vi "Main.vi"(10 "CaptureDetectionLoopDataIn":T1={"Period"=-1, "Reset"=TRUE, "Iteration"=0, "Capture"=path "", "Mode"={"Replay"=enum."None", "Record"=enum."None"}, "Replay Run ID"="", "Module Launched Timestamp"=timestamp(0 s since 1904-01-01), "Frame Number"=0, "Record Run ID"="", "Core Module ID"=0}, 11 "Module Admin":refnum<class "Delacor_lib_QMH_Cloneable Module Admin.lvclass">) -> ()   [LabVIEW 2026, in "UserEventRecorder.lvlib"]
doc: "This template is based off of the Queued Message Handler design pattern and the Queued Message Handler project template that ships with LabVIEW.\n\nThe main difference is that the queue is private to this module and communication between modules is performed via Broadcast and Request events.\n\nRequest events are wrapped in public API methods and are handled in the Event Handling Loop (EHL) of this VI. Any module can register for Broadcast events sent by this module. The EHL generates messages based on user interface actions.\n\nThe Message Handling Loop (MHL) processes messages generated by the EHL, or by other messages. The messages are string values, so new messages can be added easily to the Message Cases case structure in the MHL. Each message cluster can also provide an optional value for Message Data, which is a variant that can be converted to whatever message-specific data is required.\n_____\nBased on DQMH Dev Tools: Project Template 7.1.2.1547."
uses:
  UserEventRecorder.lvlib
  <vilib>/Delacor/Delacor QMH/Libraries/Cloneable Module Admin_class/Delacor_lib_QMH_Cloneable Module Admin.lvclass
  C:/Program Files/National Instruments/LabVIEW 2026/vi.lib/Delacor/Delacor QMH/Libraries/Module Admin_class/Delacor_lib_QMH_Module Admin.lvclass
  Launcher/Capture detection loop data--cluster.ctl
  Launcher/Mode.ctl
  ReplayMode.ctl
  RecordMode.ctl
  <vilib>/Wovalab/Utilities/Helper Loop Periodic Timing/Late Execution Mode--enum.ctl
  <vilib>/Wovalab/Utilities/Helper Loop Periodic Timing/Helper Loop Periodic Timing.lvclass/Helper Loop Periodic Timing.ctl
  Module Data--cluster.ctl
  <vilib>/Delacor/Delacor QMH/Libraries/Message Queue_class/Delacor_lib_QMH_Message Queue.lvclass/Delacor_lib_QMH_Message Queue.ctl
  <vilib>/Delacor/Delacor QMH/Libraries/Cloneable Module Admin_class/Delacor_lib_QMH_Cloneable Module Admin.lvclass/Delacor_lib_QMH_Cloneable Module Admin.ctl
  Stop Argument--cluster.ctl
  <vilib>/Delacor/Delacor QMH/Libraries/Module Admin_class/Delacor_lib_QMH_Module Admin.lvclass/Delacor_lib_QMH_Module Admin.ctl
  User Events Metadata.ctl
  <vilib>/Utility/miscctls.llb/LVPointTypeDef.ctl
  2c07e02c-bc34-4e84-878d-ebcb2aa1d67e.vi
  a20b1bd1-d842-476b-b4b8-d722f44d1f2b.vi
  <vilib>/Delacor/Delacor QMH/Libraries/Message Queue_class/Delacor_lib_QMH_Enqueue Message (Single).vi
  <vilib>/Delacor/Delacor QMH/Libraries/Cloneable Module Admin_class/Delacor_lib_QMH_Get Module ID.vi
  <vilib>/Delacor/Delacor QMH/Libraries/Module Admin_class/Delacor_lib_QMH_Get External Launch.vi
  <vilib>/Wovalab/Utilities/Helper Loop Periodic Timing/Stop Helper Loop Internal.vi
  <vilib>/Wovalab/Utilities/Helper Loop Periodic Timing/U32 Max Value--constant.vi
  <vilib>/Wovalab/Utilities/Helper Loop Periodic Timing/Update Last Execution Time.vi
  <vilib>/Wovalab/Utilities/Helper Loop Periodic Timing/Loops Events AE.vi
  <vilib>/Wovalab/Utilities/Helper Loop Periodic Timing/Notify Monitoring Window.vi
  <vilib>/Wovalab/Utilities/Helper Loop Periodic Timing/Monitoring--global.vi
  <userlib>/_OpenG.lib/comparison/comparison.llb/U32 Changed__ogtk.vi
  <vilib>/JDP Science/JSONtext/Variant to JSON Text.vi
  <vilib>/Wovalab/Utilities/Helper Loop Periodic Timing/Helper Loop Periodic Timing.lvclass
  <vilib>/JDP Science/JSONtext/LVClass Serializer/JSONtext LVClass Serializer.lvclass
  <vilib>/Delacor/Delacor QMH/Libraries/Message Queue_class/Delacor_lib_QMH_Message Queue.lvclass
  Launcher/Launcher.lvlib
  User32.dll
  <userlib>/_OpenG.lib/comparison/comparison.llb/openg_comparison__ogtk.lvlib
panel:
  out "Deficit":u32
  out "Frame Number":u32
  out "element 2":i32
  out "element":i32
  out "x != 0? 2":bool
  out "x != 0?":bool
  out "error out":errorcluster
  out "Status":string
  in  "Simulate EHL Error":bool
  in  "Simulate MHL Error":bool
  # "Other processes communicate with this Module via its Public API (wrappers for its Request Events).\n\nThis Module communicates with other processes via its Broadcast Events.\nAny process that wants to receive these messages can register for this module's Broadcast events."
  # "This template is for the DQMH framework. See the block diagram for more information on how to use this template."
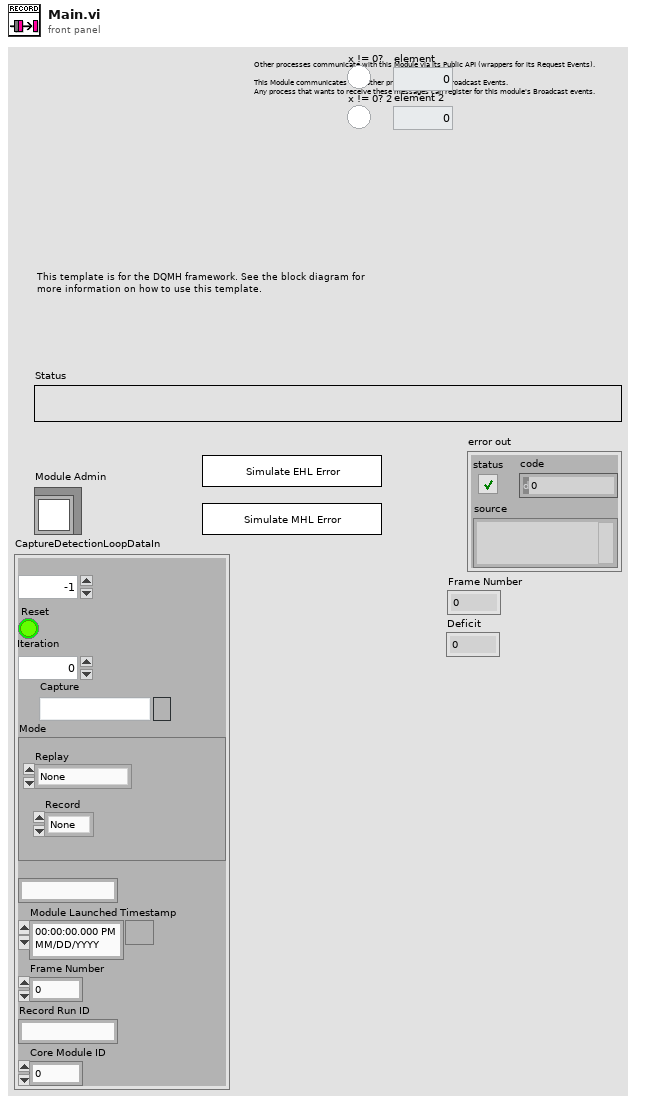
[diagram p1: front panel]
types:
  T1 = typedef "Capture detection loop data--cluster.ctl" = cluster{"Period":i32, "Reset":bool, "Iteration":i32, "Capture":path, "Mode":T2, "Replay Run ID":string, "Module Launched Timestamp":timestamp, "Frame Number":u32, "Record Run ID":string, "Core Module ID":i32}
  T2 = typedef "Mode.ctl" = cluster{"Replay":T3, "Record":T4}
  T3 = typedef "ReplayMode.ctl" = enum16{"None", "User Events"}
  T4 = typedef "RecordMode.ctl" = enum16{"None", "User Events", "Benchmarks", "User Events and Benchmarks"}
  T5 = typedef "Wovalab_lib_Utilities.lvlib/Helper Loop Periodic Timing.lvclass/Late Execution Mode--enum.ctl" = enum16{"No change", "Process missed periods ignoring original phase", "Process missed periods maintaining original phase"}
  T6 = typedef "UserEventRecorder.lvlib/Request Events--cluster.ctl" = cluster{"Stop Module":refnum<user-event>, "Show Panel":refnum<user-event>, "Hide Panel":refnum<user-event>, "Show Diagram":refnum<user-event>, "Get Module Execution Status":refnum<user-event>, "Record Frame Mouse Metadata":refnum<user-event>}
  T7 = typedef "Launcher.lvlib/Broadcast Events--cluster.ctl" = cluster{"Module Did Init":refnum<user-event>, "Status Updated":refnum<user-event>, "Error Reported":refnum<user-event>, "Module Did Stop":refnum<user-event>, "Update Module Execution Status":refnum<user-event>, "Start Capture Detection Loop":refnum<user-event>, "Benchmark Started":refnum<user-event>, "Broadcast number of frames and run ID":refnum<user-event>}
  T8 = typedef "UserEventRecorder.lvlib/Module Data--cluster.ctl" = cluster{"Status":string}
  T9 = typedef "User Events Metadata.ctl" = cluster{"Cursor Position X":i32, "Cursor Position Y":i32, "Left Button Click":bool, "Right Button Click":bool, "Frame Number":u32}
  T10 = enum16{"open", "replace", "create", "open or create", "replace or create", "replace or create with confirmation"}
  T11 = enum32{"invalid lock state", "Not Locked", "Locked (No Password)", "Password-protected"}
  T12 = typedef "UserEventRecorder.lvlib/Stop Argument--cluster.ctl" = cluster{"Module ID":i32, "Origin":string, "Exit via Stop Module Req?":bool, "Wait for Module to stop?":bool}
  T13 = typedef "LVPointTypeDef.ctl" = cluster{"Horizontal":i16, "Vertical":i16}
  T14 = enum32{"Invalid", "Standard", "Closed", "Hidden", "Minimized", "Maximized"}
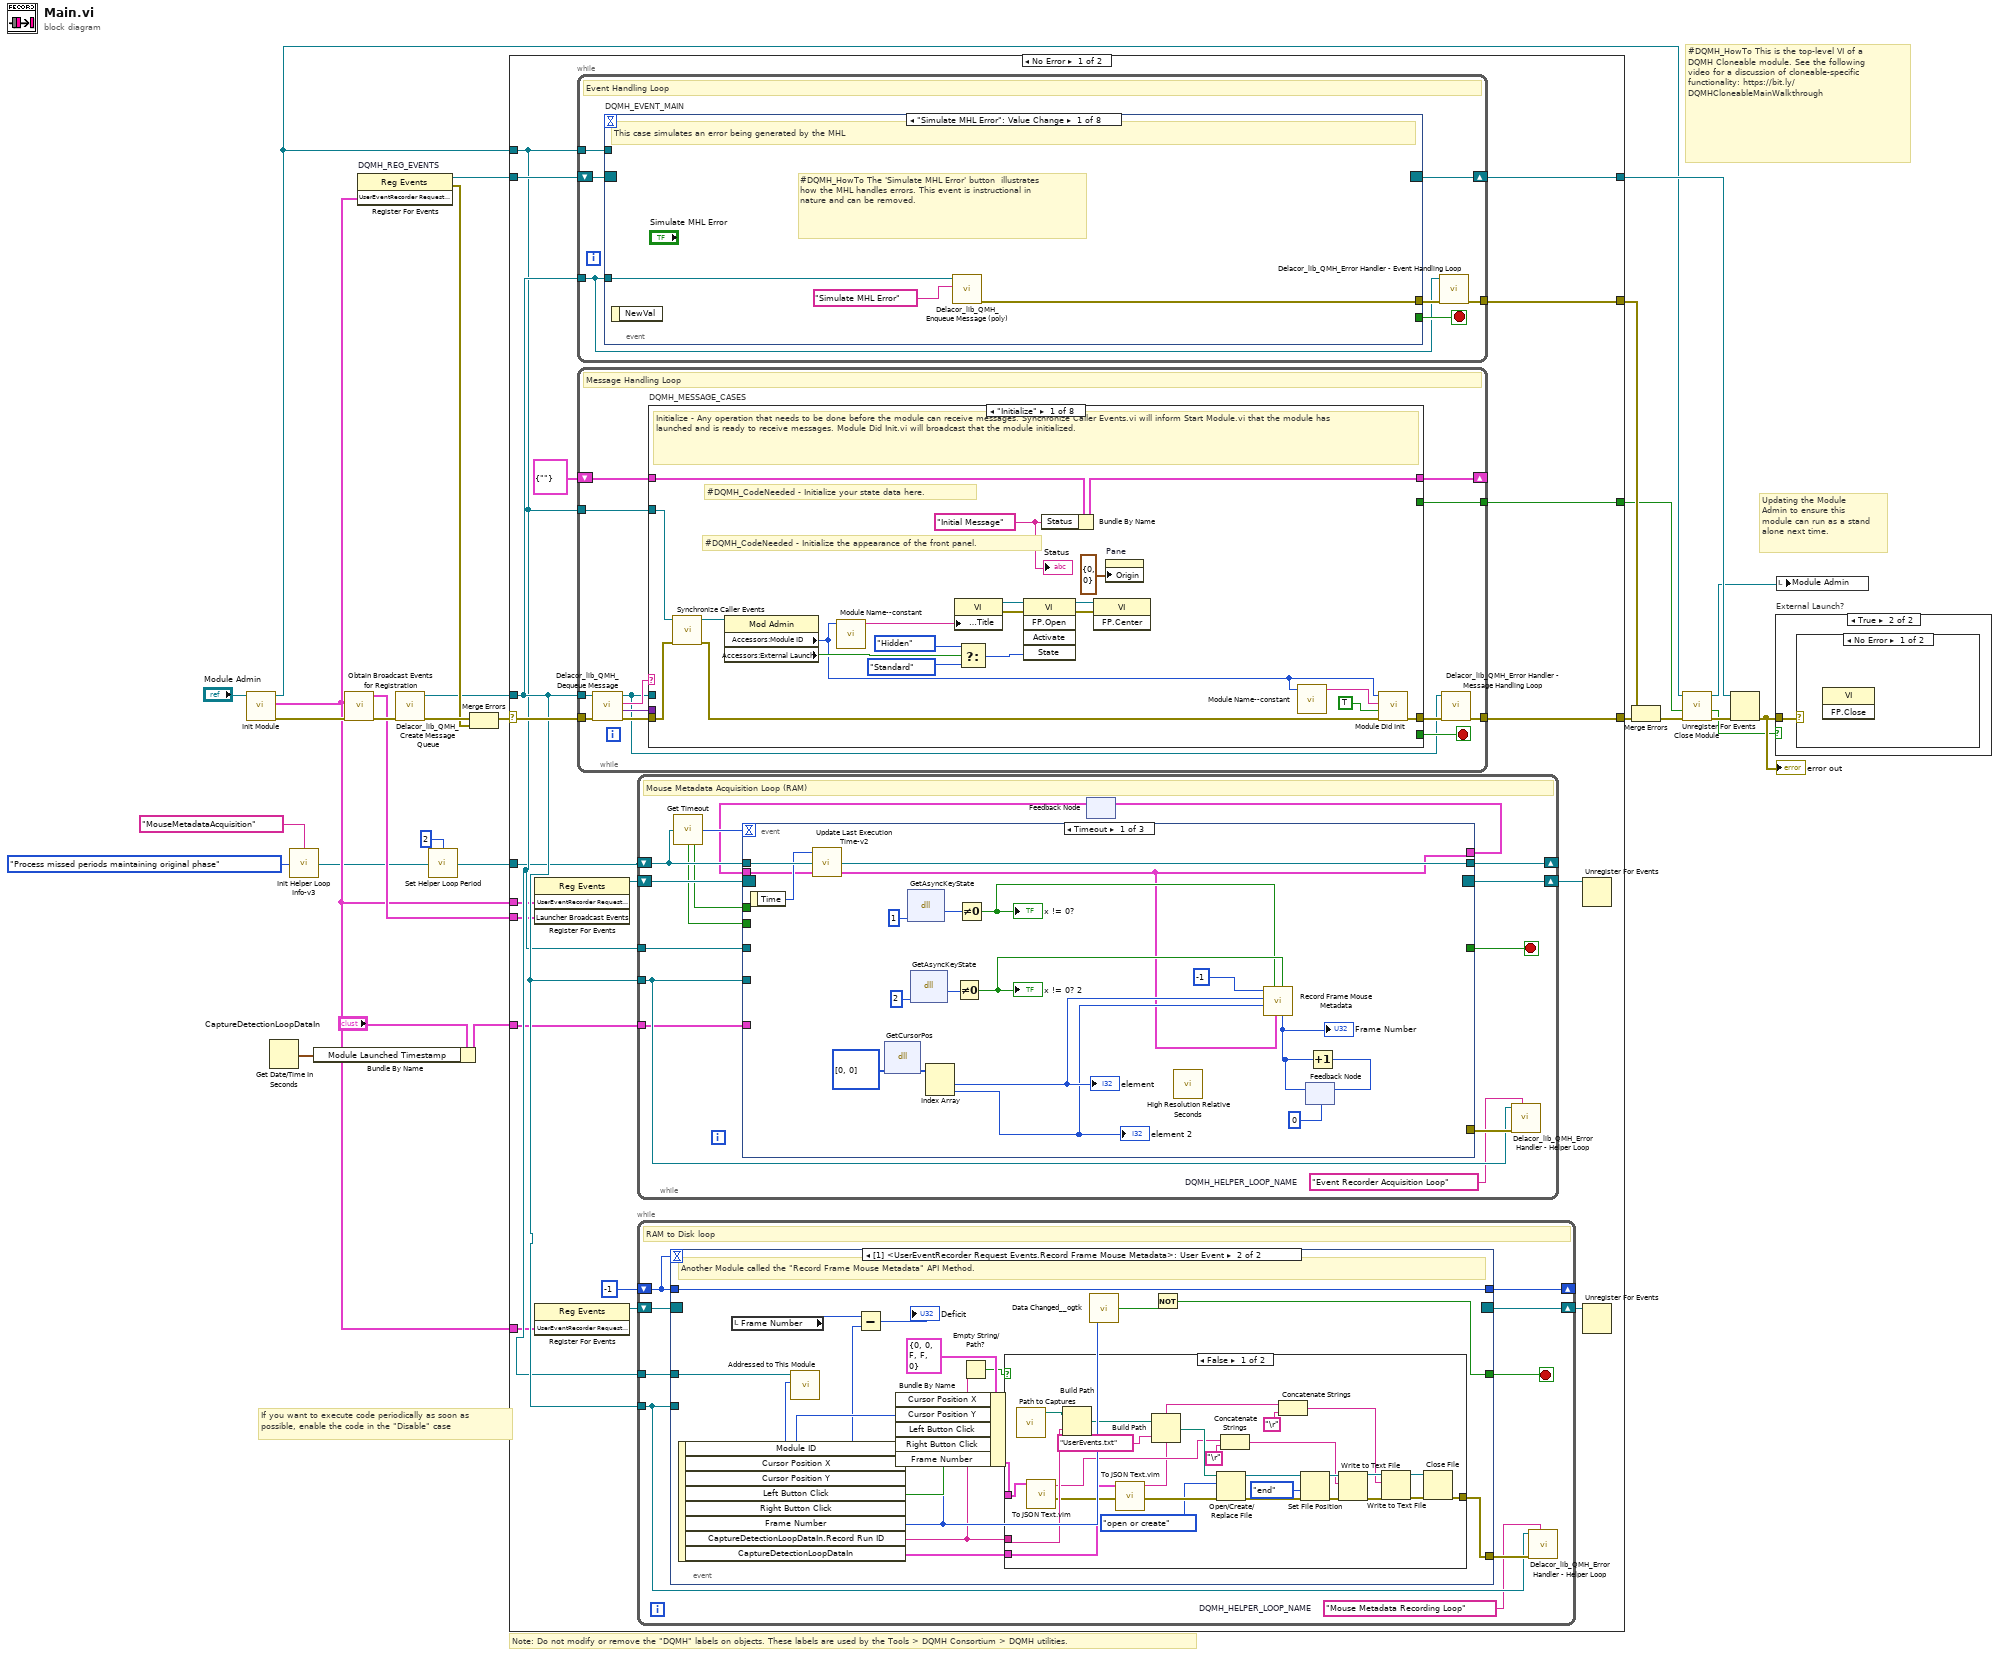
[diagram p0: block diagram]
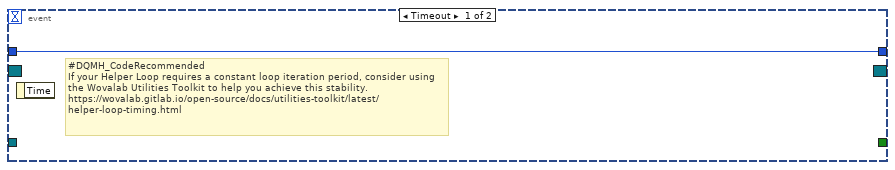
[diagram p2: hidden frame]
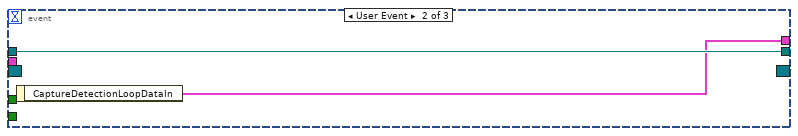
[diagram p4: hidden frame]
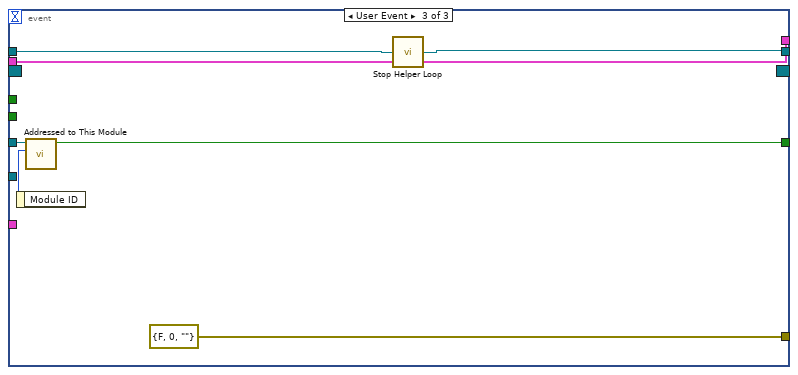
[diagram p5: hidden frame]
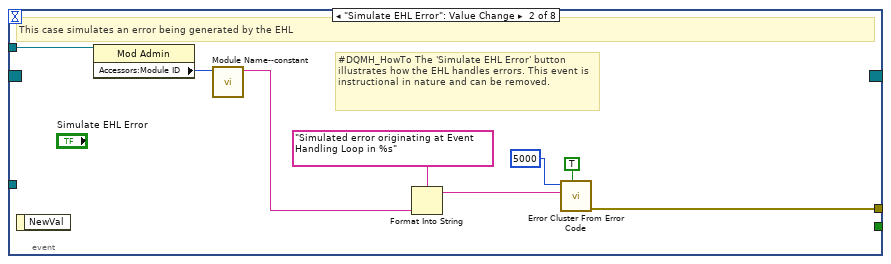
[diagram p6: hidden frame]
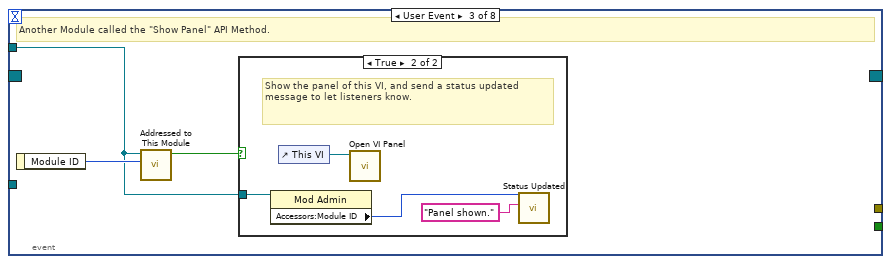
[diagram p7: hidden frame]
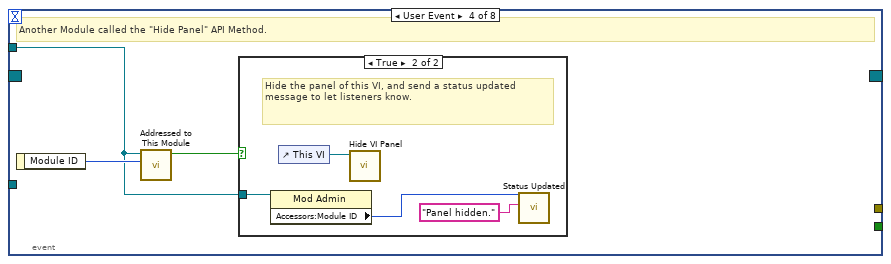
[diagram p9: hidden frame]
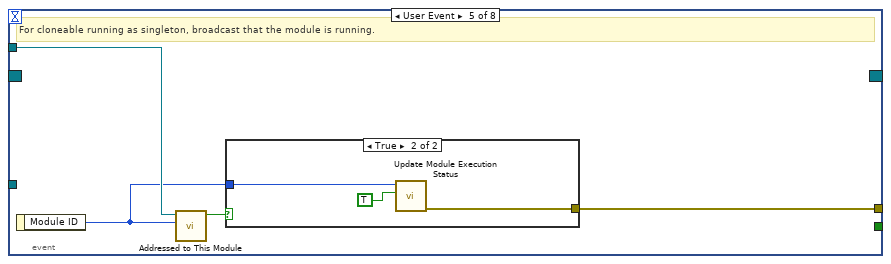
[diagram p11: hidden frame]
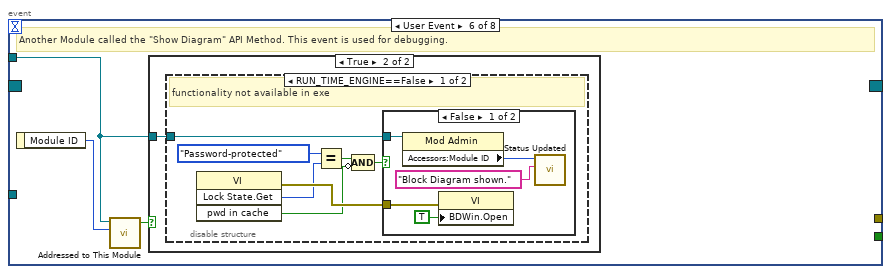
[diagram p13: hidden frame]
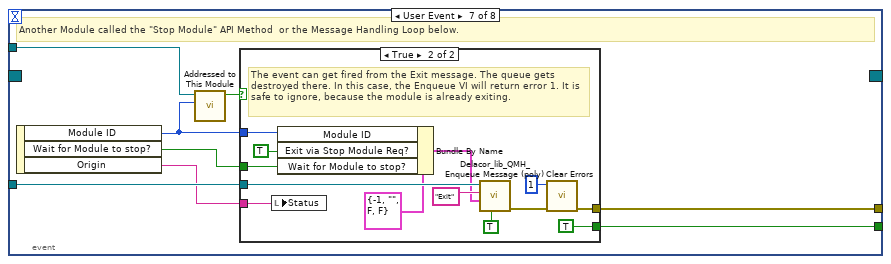
[diagram p17: hidden frame]
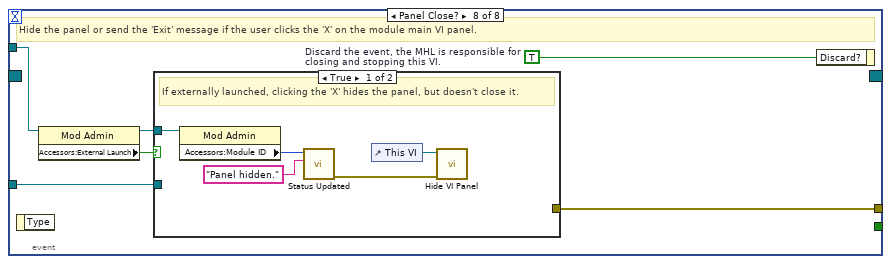
[diagram p19: hidden frame]
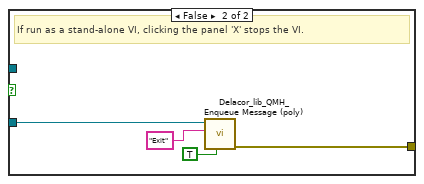
[diagram p20: hidden frame]
diagram:
  # "If you want to execute code periodically as soon as possible, enable the code in the \"Disable\" case"
  # "#DQMH_HowTo This is the top-level VI of a DQMH Cloneable module. See the following video for a discussion of cloneable-specific functionality: https://bit.ly/DQMHCloneableMainWalkthrough"
  # "Note: Do not modify or remove the \"DQMH\" labels on objects. These labels are used by the Tools > DQMH Consortium > DQMH utilities."
  # "Updating the Module Admin to ensure this module can run as a stand alone next time."
  n1 = call "Init Module.vi"("Cloneable Module Admin in"="Module Admin") -> ("error out"=w12:errorcluster, "UserEventRecorder Request Events"=w9:T6, "Cloneable Module Admin out"=w16:refnum<class "Delacor_lib_QMH_Cloneable Module Admin.lvclass">)  [unwired: 8 in]
  n2 = Get Date/Time In Seconds() -> (seconds since 1Jan1904=w1:timestamp)
  n3 = call <vilib>:"Init Helper Loop Info-v3.vi"("Late Execution Mode (Process missed periods ignoring original phase)"=Late_Execution_Mode--enum."Process missed periods maintaining original phase", "Loop Name (\"\": Caller VI)"="MouseMetadataAcquisition" ("Loop Name (\"\": Caller VI)")) -> ("Helper Loop Periodic Timing"=w5:refnum<class "Helper Loop Periodic Timing.lvclass">)
  n4 = Bundle By Name(cluster="CaptureDetectionLoopDataIn", "Module Launched Timestamp"=w1) -> (w2:T1)
  n5 = call "Obtain Broadcast Events for Registration.vi"("error in"=w12) -> ("error out"=w11:errorcluster, "Launcher Broadcast Events"=w10:T7)  [unwired: 8 in, 1 out]
  n6 = register-events "DQMH_REG_EVENTS"(w9) -> (reference out=w19:refnum<event-registration>, error out=w21:errorcluster)  [unwired: 2 in]
  n7 = call <vilib>:"Delacor_lib_QMH_Create Message Queue.vi"("error in"=w11) -> ("error out"=w23:errorcluster, "Message Queue"=w18:refnum<class "Delacor_lib_QMH_Message Queue.lvclass">)  [unwired: 9 in]
  n8 = call <vilib>:"Set Helper Loop Period.vi"("Period (ms)"=2, "Helper Loop Periodic Timing in"=w5) -> ("Helper Loop Periodic Timing out"=w4:refnum<class "Helper Loop Periodic Timing.lvclass">)  [unwired: 13 in]
  n9 = Merge Errors(w23, w21) -> (w22:errorcluster)
  n10 = case shown="No Error" w22 {
    selector: w22 -> [w45 w342]
    tunnel: [w47 w341] -> w26
    tunnel: [w44 w340] -> w20
    tunnel: w19 -> [w42 w340]
    tunnel: w18 -> [w41 w333]
    tunnel: [w46 _] -> w27
    tunnel: w16 -> [w40 w336]
    tunnel: [w39 _] -> w14
    tunnel: w9 -> [w38 _]
    tunnel: w10 -> [w35 _]
    tunnel: w9 -> [w34 _]
    tunnel: w4 -> [w30 _]
    tunnel: w2 -> [w29 _]
    frame No Error {
      n11 = register-events ("DQMH_HELPER_REGFOREVENTS")(w38, w35) -> (reference out=w36:refnum<event-registration>)  [unwired: 2 in, 1 out]
      n12 = register-events ("DQMH_HELPER_REGFOREVENTS")(w34) -> (reference out=w32:refnum<event-registration>)  [unwired: 2 in, 1 out]
      n13 = while {
        tunnel: w41 -> [w143]
        shift-right: [w146] -> w44
        shift-left: w42 -> [w147]
        tunnel: [w148] -> w46
        tunnel: w40 -> [w144]
        stop <- w145 stop-if-true
        # "Event Handling Loop"
        n14 = event "DQMH_EVENT_MAIN" shown="[0] \"Simulate MHL Error\": Value Change" {
          selector: w147 -> [_ _ _ _ _ _ _ _]
          dyn-events: [_ _ _ _ _ _ _ _] -> w146
          timeout: _ -> [_ _ _ _ _ _ _ _]
          tunnel: [_ _ _ _ _ _ w201 _] -> w145
          tunnel: w143 -> [w151 _ _ _ _ _ w204 w221]
          tunnel: [w152 w160 _ _ w178 _ w205 w224] -> w149
          tunnel: w144 -> [_ w159 w161 w168 w176 w182 w203 w222]
          event "Simulate MHL Error": Value Change {
            # "#DQMH_HowTo The 'Simulate MHL Error' button  illustrates how the MHL handles errors. This event is instructional in nature and can be removed."
            # "This case simulates an error being generated by the MHL"
            n15 = event-data() -> ()  [unwired: 1 in, 1 out]
            n16 = call-poly <vilib>:"Delacor_lib_QMH_Enqueue Message (poly).vi"("Message"="Simulate MHL Error", "Message Queue in"=w151) -> ("error out"=w152:errorcluster)  [unwired: 8 in, 1 out]
          }
          event "Simulate EHL Error": Value Change {
            # "#DQMH_HowTo The 'Simulate EHL Error' button  illustrates how the EHL handles errors. This event is instructional in nature and can be removed."
            # "This case simulates an error being generated by the EHL"
            n17 = event-data() -> ()  [unwired: 1 in, 1 out]
            n18 = property on="Property Node" class="Mod Admin"(reference=w159) -> ("Accessors:Module ID"=w158:i32)  [unwired: 1 in, 2 out]
            n19 = call "Module Name--constant.vi"("Module ID"=w158) -> ("Module Name"=w153:string)  [unwired: 10 in]
            n20 = Format Into String(format string="Simulated error originating at Event Handling Loop in %s", w153) -> (resulting string=w156:string)  [unwired: 2 in, 1 out]
            n21 = call <vilib>:"Error Cluster From Error Code.vi"("show call chain? (False)"=TRUE, "error message (\"\")"=w156, "error code (0)"=5000) -> ("error out"=w160:errorcluster)  [unwired: 6 in]
          }
          event User Event {
            # "Another Module called the \"Show Panel\" API Method."
            n22 = event-data() -> ("Module ID"=w162:i32)  [unwired: 1 in]
            n23 = call "Addressed to This Module.vi"("Module ID from Argument"=w162, "Module Admin"=w161) -> ("Addressed to this instance?"=w163:bool)  [unwired: 8 in, 1 out]
            n24 = case shown="True" w163 {
              tunnel: w161 -> [_ w165]
              frame False {
              }
              frame True {
                # "Show the panel of this VI, and send a status updated message to let listeners know."
                n25 = property on="Property Node" class="Mod Admin"(reference=w165) -> ("Accessors:Module ID"=w164:i32)  [unwired: 1 in, 2 out]
                n26 = control-ref of="This VI"() -> (w167:refnum<vi>)
                n27 = call "Open VI Panel.vi"("VI"=w167) -> ()  [unwired: 10 in, 1 out]
                n28 = call "Status Updated.vi"("Status"="Panel shown." ("format string"), "Module ID"=w164) -> ()  [unwired: 9 in, 1 out]
              }
            }
          }
          event User Event {
            # "Another Module called the \"Hide Panel\" API Method."
            n29 = event-data() -> ("Module ID"=w169:i32)  [unwired: 1 in]
            n30 = call "Addressed to This Module.vi"("Module ID from Argument"=w169, "Module Admin"=w168) -> ("Addressed to this instance?"=w170:bool)  [unwired: 8 in, 1 out]
            n31 = case shown="True" w170 {
              tunnel: w168 -> [_ w172]
              frame False {
              }
              frame True {
                # "Hide the panel of this VI, and send a status updated message to let listeners know."
                n32 = property on="Property Node" class="Mod Admin"(reference=w172) -> ("Accessors:Module ID"=w171:i32)  [unwired: 1 in, 2 out]
                n33 = control-ref of="This VI"() -> (w174:refnum<vi>)
                n34 = call "Hide VI Panel.vi"("VI"=w174) -> ()  [unwired: 10 in, 1 out]
                n35 = call "Status Updated.vi"("Status"="Panel hidden." ("format string"), "Module ID"=w171) -> ()  [unwired: 9 in, 1 out]
              }
            }
          }
          event User Event {
            # "For cloneable running as singleton, broadcast that the module is running."
            n36 = event-data() -> ("Module ID"=w175:i32)  [unwired: 1 in]
            n37 = call "Addressed to This Module.vi"("Module ID from Argument"=w175, "Module Admin"=w176) -> ("Addressed to this instance?"=w177:bool)  [unwired: 8 in, 1 out]
            n38 = case shown="True" w177 {
              tunnel: [_ w181] -> w178
              tunnel: w175 -> [_ w180]
              frame False {
              }
              frame True {
                n39 = call "Update Module Execution Status.vi"("Running?"=TRUE, "Module ID"=w180) -> ("error out"=w181:errorcluster)  [unwired: 9 in]
              }
            }
          }
          event User Event {
            # "Another Module called the \"Show Diagram\" API Method. This event is used for debugging."
            n40 = event-data() -> ("Module ID"=w183:i32)  [unwired: 1 in]
            n41 = call "Addressed to This Module.vi"("Module ID from Argument"=w183, "Module Admin"=w182) -> ("Addressed to this instance?"=w184:bool)  [unwired: 8 in, 1 out]
            n42 = case shown="True" w184 {
              tunnel: w182 -> [_ w185]
              frame False {
              }
              frame True {
                n43 = disable-structure shown="RUN_TIME_ENGINE==False" {
                  disable-tunnel: w185 -> [w186 _]
                  frame condition #0 (active) {
                    # "functionality not available in exe"
                    n44 = invoke on="Invoke Node" class="VI" method="Lock State.Get"() -> (error out=w192:errorcluster, "Get Lock State"=w191:T11, "pwd in cache"=w188:bool)  [unwired: 4 in, 1 out]
                    n45 = Equal?(x=T11."Password-protected", y=w191) -> (x = y?=w189:bool)
                    n46 = Compound Arithmetic op=AND(w189, invert w188) -> (w187:bool)
                    n47 = case shown="False" w187 {
                      tunnel: w192 -> [w197 _]
                      tunnel: w186 -> [w194 _]
                      frame False {
                        n48 = property on="Property Node" class="Mod Admin"(reference=w194) -> ("Accessors:Module ID"=w193:i32)  [unwired: 1 in, 2 out]
                        n49 = property on="Property Node" class="VI"(error in=w197, "BDWin.Open"=TRUE ("Block Diagram Window:Open")) -> ()  [unwired: 1 in, 2 out]
                        n50 = call "Status Updated.vi"("Status"="Block Diagram shown." ("format string"), "Module ID"=w193) -> ()  [unwired: 9 in, 1 out]
                      }
                      frame True {
                        # "Password-protected VI, and the password is not in the cache. Do not show the diagram."
                      }
                    }
                  }
                  frame condition #1 {
                  }
                }
              }
            }
          }
          event User Event {
            # "Another Module called the \"Stop Module\" API Method  or the Message Handling Loop below."
            n51 = event-data() -> ("Module ID"=w199:i32, "Wait for Module to stop?"=w200:bool, "Origin"=w198:string)  [unwired: 1 in]
            n52 = call "Addressed to This Module.vi"("Module ID from Argument"=w199, "Module Admin"=w203) -> ("Addressed to this instance?"=w202:bool)  [unwired: 8 in, 1 out]
            n53 = case shown="True" w202 {
              tunnel: [_ w217] -> w205
              tunnel: w204 -> [_ w213]
              tunnel: [_ TRUE] -> w201
              tunnel: w200 -> [_ w208]
              tunnel: w199 -> [_ w210]
              tunnel: w198 -> [_ w206]
              frame False {
              }
              frame True {
                # "The event can get fired from the Exit message. The queue gets destroyed there. In this case, the Enqueue VI will return error 1. It is safe to ignore, because the module is already exiting."
                n54 = local write "Status"(w206) -> ()
                n55 = Bundle By Name(cluster=T12 {"Module ID"=-1, "Origin"="", "Exit via Stop Module Req?"=FALSE, "Wait for Module to stop?"=FALSE} ("Stop Argument"), "Module ID"=w210, "Exit via Stop Module Req?"=TRUE, "Wait for Module to stop?"=w208) -> (w207:T12)
                n56 = call-poly <vilib>:"Delacor_lib_QMH_Enqueue Message (poly).vi"("Priority Message? (F)"=TRUE, "Message Data"=w207, "Message"="Exit", "Message Queue in"=w213) -> ("error out"=w218:errorcluster)  [unwired: 6 in, 1 out]
                n57 = call <vilib>:"Clear Errors.vi"("error in (no error)"=w218, "specific error code to clear (0: all)"=1) -> ("error out"=w217:errorcluster)  [unwired: 4 in, 1 out]
              }
            }
          }
          event Panel Close? {
            w223 = TRUE  # Discard the event, the MHL is responsible for closing and stopping this VI.
            # "Hide the panel or send the 'Exit' message if the user clicks the 'X' on the module main VI panel."
            n58 = event-data() -> ()  [unwired: 1 in, 1 out]
            n59 = property on="Property Node" class="Mod Admin"(reference=w222) -> (reference out=w219:refnum<class "Delacor_lib_QMH_Cloneable Module Admin.lvclass">, "Accessors:External Launch"=w220:bool)  [unwired: 1 in, 1 out]
            n60 = case shown="True" w220 {
              tunnel: w221 -> [_ w232]
              tunnel: [_ w233] -> w224
              tunnel: w219 -> [w227 _]
              frame True {
                # "If externally launched, clicking the 'X' hides the panel, but doesn't close it."
                n61 = property on="Property Node" class="Mod Admin"(reference=w227) -> ("Accessors:Module ID"=w226:i32)  [unwired: 1 in, 2 out]
                n62 = call "Status Updated.vi"("Status"="Panel hidden." ("format string"), "Module ID"=w226) -> ("error out"=w225:errorcluster)  [unwired: 9 in]
                n63 = control-ref of="This VI"() -> (w229:refnum<vi>)
                n64 = call "Hide VI Panel.vi"("error in"=w225, "VI"=w229) -> ()  [unwired: 9 in, 1 out]
              }
              frame False {
                # "If run as a stand-alone VI, clicking the panel 'X' stops the VI."
                n65 = call-poly <vilib>:"Delacor_lib_QMH_Enqueue Message (poly).vi"("Priority Message? (F)"=TRUE, "Message"="Exit", "Message Queue in"=w232) -> ("error out"=w233:errorcluster)  [unwired: 7 in, 1 out]
              }
            }
            n66 = event-data ("Event Filter Node")("Discard?"=w223) -> ()  [unwired: 1 in, 1 out]
          }
        }
        n67 = call-dynamic "Delacor_lib_QMH_Error Handler - Event Handling Loop.vi"("error in"=w149, "Message Queue in"=w143) -> ("dup error in"=w148:errorcluster)  [unwired: 8 in, 1 out]
      }
      n68 = while {
        tunnel: w41 -> [w234]
        shift-right: [w241] -> _
        shift-left: T8 {"Status"=""} ("Data Cluster") -> [w242]
        tunnel: w45 -> [w245]
        tunnel: [w243] -> w47
        tunnel: w40 -> [w236]
        tunnel: [w235] -> w39
        stop <- w240 stop-if-true
        # "Message Handling Loop"
        n69 = call-dynamic "Delacor_lib_QMH_Dequeue Message.vi"("error in"=w245, "Message Queue in"=w234) -> ("error out"=w244:errorcluster, "Message Data"=w238:variant, "Message"=w239:string, "Message Queue out"=w237:refnum<class "Delacor_lib_QMH_Message Queue.lvclass">)  [unwired: 6 in]
        n70 = case "DQMH_MESSAGE_CASES" shown="\"Initialize\"" w239 {
          selector: w239 -> [_ _ _ _ _ _ _ w322]
          tunnel: w237 -> [_ _ _ _ w277 _ w314 _]
          tunnel: w244 -> [w265 w269 w272 w274 w286 w303 w320 w331]
          tunnel: [w263 w269 w271 w274 w282 w302 w315 w332] -> w246
          tunnel: w242 -> [w256 w268 w270 w273 w281 w300 w313 w329]
          tunnel: [w255 w268 w270 w273 w281 w300 w313 w329] -> w241
          tunnel: [_ _ _ _ _ _ w312 _] -> w240
          tunnel: w238 -> [_ _ _ _ w280 _ w310 _]
          tunnel: w236 -> [w251 _ _ _ w279 w298 w305 w328]
          tunnel: [_ _ _ _ _ _ w308 _] -> w235
          frame "Initialize" {
            w248 = "Initial Message" ("Initial Message")
            # "#DQMH_CodeNeeded - Initialize the appearance of the front panel."
            # "#DQMH_CodeNeeded - Initialize your state data here."
            # "Initialize - Any operation that needs to be done before the module can receive messages. Synchronize Caller Events.vi will inform Start Module.vi that the module has launched and is ready to receive messages. Module Did Init.vi will broadcast that the module initialized."
            n71 = call "Synchronize Caller Events.vi"("error in"=w265, "Module Admin"=w251) -> ("error out"=w264:errorcluster, "Module Admin out"=w250:refnum<class "Delacor_lib_QMH_Cloneable Module Admin.lvclass">)  [unwired: 8 in]
            n72 = property on="Property Node" class="Mod Admin"(reference=w250) -> ("Accessors:Module ID"=w247:i32, "Accessors:External Launch"=w252:bool)  [unwired: 1 in, 2 out]
            n73 = call "Module Name--constant.vi"("Module ID"=w247) -> ("Module Name"=w260:string)  [unwired: 10 in]
            n74 = property on="Property Node" class="VI"("Front Panel.Title"=w260) -> (reference out=w262:refnum<vi>, error out=w267:errorcluster)  [unwired: 2 in]
            n75 = Select(t=T14."Hidden" ("State"), s=w252, f=T14."Standard" ("State")) -> (s? t:f=w257:T14)
            n76 = invoke on="Invoke Node" class="VI" method="FP.Open"(reference=w262, error in=w267, "State"=w257) -> (reference out=w261:refnum<vi>, error out=w266:errorcluster)  [unwired: 2 in, 3 out]
            n77 = Bundle By Name(cluster=w256, "Status"=w248) -> (w255:T8)
            n78 = invoke on="Invoke Node" class="VI" method="FP.Center"(reference=w261, error in=w266) -> ()  [unwired: 1 in, 3 out]
            n79 = property on="Pane" class="Pane"("Origin"=T13 {"Horizontal"=0, "Vertical"=0}) -> ()  [unwired: 2 in, 2 out]
            n80 = call "Module Name--constant.vi"("Module ID"=w247) -> ("Module Name"=w253:string)  [unwired: 10 in]
            n81 = call "Module Did Init.vi"("error in"=w264, "Initialized?"=TRUE, "Origin"=w253, "Module ID"=w247) -> ("error out"=w263:errorcluster)  [unwired: 7 in]
            "Status" <- w248
          }
          frame "---Module Specific---" {
            # "Separator -- The following cases handle messages specific to this Module."
          }
          frame "---Copy This Frame---" {
            # "Duplicate this frame when creating new messages.  Change this comment in the duplicated frame to describe this message."
            n82 = Merge Errors(w272) -> (w271:errorcluster)
          }
          frame "---Exit and Error Handling---" {
            # "Separator - the following cases handle errors and exit messages."
          }
          frame "Error" {
            # "#DQMH_CodeRecommended - If the module is running in standalone mode (External Launch = FALSE), this code will pop up an error dialog and call the 'Exit' message if an error occurs. Add more fine-grained error management here."
            # "Error - Check the error message data and respond accordingly. This message is sent by the \"Error Handler\" VIs at the end of each loop in this application."
            n83 = property on="Property Node" class="Mod Admin"(reference=w279) -> ("Accessors:External Launch"=w278:bool, "Accessors:Module ID"=w276:i32)  [unwired: 1 in, 2 out]
            n84 = Variant To Data(error in=w286, type=errorcluster {"status"=FALSE, "code"=0, "source"=""} ("error constant"), Variant=w280) -> (data=w275:errorcluster, error out=w284:errorcluster)
            n85 = local write "error out"(w275) -> ()
            n86 = call "Error Reported.vi"("Error"=w275, "Module ID"=w276) -> ()  [unwired: 9 in, 1 out]
            n87 = case shown="False" w278 {
              tunnel: [w291 _] -> w283
              tunnel: w277 -> [w289 _]
              tunnel: w275 -> [w290 _]
              frame False {
                n88 = disable-structure shown="Default" {
                  disable-tunnel: w290 -> [w292 _]
                  frame condition #0 (active) {
                    # "If the module is running standalone, then pop up an error dialog and call the \"Exit\" message."
                    n89 = call <vilib>:"Simple Error Handler.vi"("error in (no error)"=w292) -> ()  [unwired: 4 in, 5 out]
                  }
                  frame condition #1 {
                    # "To prevent the Simple Error Handler VI from being loaded (e.g. when deploying to a Real-Time target), add the Conditional Disable Symbol \"DQMH_Disable_SEH\" to your project and set it to TRUE."
                  }
                }
                n90 = call-poly <vilib>:"Delacor_lib_QMH_Enqueue Message (poly).vi"("Priority Message? (F)"=TRUE, "Message"="Exit", "Message Queue in"=w289) -> ("error out"=w291:errorcluster)  [unwired: 7 in, 1 out]
              }
              frame True {
                # "If the module was launched externally, calling the Error Reported broadcast VI is the only action performed by the \"Error\" message. The module's caller can then process the error appropriately."
              }
            }
            n91 = Merge Errors(w284, w283) -> (w282:errorcluster)
          }
          frame "Simulate MHL Error" {
            # "#DQMH_HowTo The 'Simulate MHL Error' button  illustrates how the MHL handles errors. This event is instructional in nature and can be removed."
            # "Simulate an error occurring at the MHL"
            n92 = property on="Property Node" class="Mod Admin"(reference=w298) -> ("Accessors:Module ID"=w299:i32)  [unwired: 1 in, 2 out]
            n93 = call "Module Name--constant.vi"("Module ID"=w299) -> ("Module Name"=w294:string)  [unwired: 10 in]
            n94 = Format Into String(format string="Simulated error originating at Message Handling Loop in %s", w294) -> (resulting string=w295:string)  [unwired: 2 in, 1 out]
            n95 = call <vilib>:"Error Cluster From Error Code.vi"("show call chain? (False)"=TRUE, "error message (\"\")"=w295, "error code (0)"=5001) -> ("error out"=w301:errorcluster)  [unwired: 6 in]
            n96 = Merge Errors(w303, w301) -> (w302:errorcluster)
          }
          frame "Exit" {
            w311 = 91  # 91: not all Exit messages will have an argument
            w312 = TRUE  # Stop the VI
            # "Release the message queue reference"
            # "#DQMH_CodeNeeded - Add any required cleanup code here."
            # "Exit - Exit the application."
            n97 = Variant To Data(error in=w320, type=T12 {"Module ID"=-1, "Origin"="", "Exit via Stop Module Req?"=FALSE, "Wait for Module to stop?"=FALSE} ("Stop Argument"), Variant=w310) -> (data=w307:T12, error out=w316:errorcluster)
            n98 = call <vilib>:"Clear Errors.vi"("error in (no error)"=w316, "specific error code to clear (0: all)"=w311) -> ("error out"=w319:errorcluster)  [unwired: 4 in, 1 out]
            n99 = property on="Property Node" class="Mod Admin"(reference=w305) -> ("Accessors:Module ID"=w304:i32)  [unwired: 1 in, 2 out]
            n100 = control-ref of="This VI"() -> (w306:refnum<vi>)
            n101 = call-dynamic "Delacor_lib_QMH_Release Message Queue.vi"("error in"=w319, "Message Queue"=w314) -> ("error out"=w318:errorcluster)  [unwired: 9 in]
            n102 = call "Handle Exit.vi"("Stop Argument"=w307, "Module Admin in"=w305, "VI reference"=w306) -> ("error out"=w317:errorcluster, "Wait for Stop?"=w308:bool)  [unwired: 7 in]
            n103 = Merge Errors(w318, w317) -> (w315:errorcluster)
            n104 = call "Error Reported.vi"("Error"=w315, "Module ID"=w304) -> ()  [unwired: 9 in, 1 out]
          }
          frame Default {
            # "'Default' case only runs if there is a message that isn't defined in any of the other cases.  Output a programming error."
            n105 = property on="Property Node" class="Mod Admin"(reference=w328) -> ("Accessors:Module ID"=w327:i32)  [unwired: 1 in, 2 out]
            n106 = call "Module Name--constant.vi"("Module ID"=w327) -> ("Module Name"=w321:string)  [unwired: 10 in]
            n107 = Format Into String(format string="The invalid message string \"%s\" was received in the Message Handling Loop for module \"%s\".", w322, w321) -> (resulting string=w324:string)  [unwired: 2 in, 1 out]
            n108 = call <vilib>:"Error Cluster From Error Code.vi"("show call chain? (False)"=TRUE, "error message (\"\")"=w324, "error code (0)"=1) -> ("error out"=w330:errorcluster)  [unwired: 6 in]
            n109 = Merge Errors(w331, w330) -> (w332:errorcluster)
          }
        }
        n110 = call-dynamic "Delacor_lib_QMH_Error Handler - Message Handling Loop.vi"("error in"=w246, "Message Queue in"=w237) -> ("dup error in"=w243:errorcluster)  [unwired: 8 in, 1 out]
      }
      n111 = while "DQMH_HELPER_LOOP" {
        shift-right: [w115] -> _
        shift-left: w30 -> [w107]
        shift-right: [w113] -> w37
        shift-left: w36 -> [w114]
        tunnel: w41 -> [w110]
        tunnel: w40 -> [w108]
        tunnel: w29 -> [w103]
        stop <- w112 stop-if-true
        w109 = "Event Recorder Acquisition Loop"  # DQMH_HELPER_LOOP_NAME
        # "Mouse Metadata Acquisition Loop (RAM)"
        n112 = call <vilib>:"Get Timeout.vi"("Helper Loop Periodic Timing"=w107) -> ("Timeout (ms)"=w106:i32, "Late?"=w105:bool, "First Execution Since Period Modification?"=w104:bool)  [unwired: 12 in]
        n113 = feedback #1() -> (w101:T1)  [unwired: 1 in]
        n114 = event "DQMH_HELPER_EVENT_STRUCTURE" shown="[0] Timeout" {
          selector: w114 -> [_ _ _]
          dyn-events: [_ _ _] -> w113
          timeout: w106 -> [_ _ _]
          tunnel: w107 -> [w119 w135 w138]
          tunnel: [w118 w135 w137] -> w115
          tunnel: [_ _ w140] -> w112
          tunnel: [_ _ errorcluster {"status"=FALSE, "code"=0, "source"=""} ("error constant")] -> w111
          tunnel: w110 -> [_ _ _]
          tunnel: w108 -> [_ _ w141]
          tunnel: w105 -> [_ _ _]
          tunnel: w104 -> [_ _ _]
          tunnel: w103 -> [_ _ _]
          tunnel: [w116 w134 w136] -> w102
          tunnel: w101 -> [w116 _ w136]
          event Timeout {
            n115 = event-data() -> ("Time"=w117:u32)  [unwired: 1 in]
            n116 = call <vilib>:"Update Last Execution Time-v2.vi"("Time"=w117, "Helper Loop Periodic Timing in"=w119) -> ("Helper Loop Periodic Timing out"=w118:refnum<class "Helper Loop Periodic Timing.lvclass">)  [unwired: 12 in, 1 out]
            n117 = dll-call lib="User32.dll" fn="GetCursorPos"("Position"=i32[] [0, 0]) -> ("Position"=w132:i32[])  [unwired: 4 in, 2 out]
            n118 = dll-call lib="User32.dll" fn="GetAsyncKeyState" label="Left Button Click"("vKey"=i16 1) -> ("return type"=w129:i16)  [unwired: 4 in, 2 out]
            n119 = dll-call lib="User32.dll" fn="GetAsyncKeyState" label="Right Button Click"("vKey"=i16 2) -> ("return type"=w128:i16)  [unwired: 4 in, 2 out]
            n120 = Index Array(array=w132) -> (element #1=w124:i32, element #2=w123:i32)  [unwired: 2 in]
            "element" <- w124
            "element 2" <- w123
            n121 = Not Equal To 0?(x=w128) -> (x != 0?=w127:bool)
            "x != 0? 2" <- w127
            n122 = Not Equal To 0?(x=w129) -> (x != 0?=w126:bool)
            "x != 0?" <- w126
            n123 = call <vilib>:"High Resolution Relative Seconds.vi"() -> ()  [unwired: 1 out]
            n124 = feedback #2(u32 0 ("Frame Number")) -> (w120:u32)
            "Frame Number" <- w120
            n125 = call "Record Frame Mouse Metadata.vi"("Frame Number"=w120, "Right Button Click"=w127, "CaptureDetectionLoopDataIn"=w116, "Left Button Click"=w126, "Cursor Position Y"=w123, "Cursor Position X"=w124, "Module ID"=-1) -> ()  [unwired: 4 in, 1 out]
            n126 = Increment(x=w120) -> (x+1=w121:u32)
            n127 = feedback-in #2(w121) -> ()
          }
          event User Event {
            n128 = event-data() -> ("CaptureDetectionLoopDataIn"=w134:T1)  [unwired: 1 in]
          }
          event User Event {
            n129 = event-data() -> ("Module ID"=w139:i32)  [unwired: 1 in]
            n130 = call "Addressed to This Module.vi"("Module ID from Argument"=w139, "Module Admin"=w141) -> ("Addressed to this instance?"=w140:bool)  [unwired: 8 in, 1 out]
            n131 = call <vilib>:"Stop Helper Loop.vi"("Helper Loop Periodic Timing in"=w138) -> ("Helper Loop Periodic Timing out"=w137:refnum<class "Helper Loop Periodic Timing.lvclass">)
          }
        }
        n132 = feedback-in #1(w102) -> ()
        n133 = call-dynamic "Delacor_lib_QMH_Error Handler - Helper Loop.vi"("Error Debug"=w109, "error in"=w111, "Message Queue in"=w110) -> ()  [unwired: 7 in, 2 out]
      }
      n134 = while "DQMH_HELPER_LOOP" {
        shift-right: [w56] -> _
        shift-left: -1 -> [w55]
        shift-right: [w53] -> w33
        shift-left: w32 -> [w54]
        tunnel: w41 -> [w50]
        tunnel: w40 -> [w48]
        stop <- w52 stop-if-true
        w49 = "Mouse Metadata Recording Loop"  # DQMH_HELPER_LOOP_NAME
        # "RAM to Disk loop"
        n135 = event "DQMH_HELPER_EVENT_STRUCTURE" shown="[1] <UserEventRecorder Request Events.Record Frame Mouse Metadata>: User Event" {
          selector: w54 -> [_ _]
          dyn-events: [_ _] -> w53
          timeout: w55 -> [_ _]
          tunnel: w55 -> [w57 w75]
          tunnel: [w57 w75] -> w56
          tunnel: [_ w60] -> w52
          tunnel: [_ w72] -> w51
          tunnel: w50 -> [_ _]
          tunnel: w48 -> [_ w74]
          event Timeout {
            # "#DQMH_CodeRecommended\nIf your Helper Loop requires a constant loop iteration period, consider using the Wovalab Utilities Toolkit to help you achieve this stability.\nhttps://wovalab.gitlab.io/open-source/docs/utilities-toolkit/latest/helper-loop-timing.html"
            n136 = event-data() -> ()  [unwired: 1 in, 1 out]
          }
          event User Event {
            # "Another Module called the \"Record Frame Mouse Metadata\" API Method."
            n137 = event-data() -> ("Module ID"=w73:i32, "Cursor Position X"=w70:i32, "Cursor Position Y"=w69:i32, "Left Button Click"=w68:bool, "Right Button Click"=w67:bool, "Frame Number"=w62:u32, "CaptureDetectionLoopDataIn.Record Run ID"=w59:string, "CaptureDetectionLoopDataIn"=w65:T1)  [unwired: 1 in]
            n138 = local read "Frame Number"() -> (w64:u32)
            n139 = call "Addressed to This Module.vi"("Module ID from Argument"=w73, "Module Admin"=w74) -> ()  [unwired: 8 in, 2 out]
            n140 = Subtract(x=w64, y=w62) -> (x-y=→"Deficit":u32)
            n141 = Bundle By Name(cluster=T9 {"Cursor Position X"=0, "Cursor Position Y"=0, "Left Button Click"=FALSE, "Right Button Click"=FALSE, "Frame Number"=0} ("User Events Metadata"), "Cursor Position X"=w70, "Cursor Position Y"=w69, "Left Button Click"=w68, "Right Button Click"=w67, "Frame Number"=w62) -> (w66:T9)
            n142 = Empty String/Path?(string/path=w59) -> (empty?=w58:bool)
            n143 = case shown="False" w58 {
              tunnel: w59 -> [w100 _]
              tunnel: [w97 _] -> w72
              tunnel: w66 -> [w84 _]
              tunnel: w65 -> [w83 _]
              frame False {
                n144 = call "Path to Captures.vi"() -> ("Captures"=w96:path)  [unwired: 11 in]
                n145 = call "To JSON Text.vim"("Anything"=w84) -> ("error out"=w94:errorcluster, "<JSON>"=w92:string)  [unwired: 9 in]
                n146 = Build Path(base path=w96, name or relative path=w100) -> (appended path=w95:path)
                n147 = call "To JSON Text.vim"("Anything"=w83) -> ("<JSON>"=w76:string)  [unwired: 9 in, 1 out]
                n148 = Build Path(base path=w95, name or relative path="UserEvents.txt" ("Run ID")) -> (appended path=w98:path)
                n149 = Open/Create/Replace File(file path (use dialog)=w98, error in=w94, operation (0:open)=T10."open or create") -> (refnum out=w90:refnum<file>, error out=w89:errorcluster)  [unwired: 3 in, 1 out]
                n150 = Concatenate Strings(w92, "\r") -> (w86:string)
                n151 = Concatenate Strings(w76, "\r") -> (w77:string)
                n152 = Set File Position(refnum=w90, from (0:start)=enum16{"start", "end", "current"}."end", error in=w89) -> (refnum out=w87:refnum<file>, error out=w88:errorcluster)  [unwired: 1 in]
                n153 = Write to Text File(file (use dialog)=w87, text=w86, error in=w88) -> (refnum out=w78:refnum<file>, error out=w81:errorcluster)  [unwired: 1 in, 1 out]
                n154 = Write to Text File(file (use dialog)=w78, text=w77, error in=w81) -> (refnum out=w79:refnum<file>, error out=w80:errorcluster)  [unwired: 1 in, 1 out]
                n155 = Close File(refnum=w79, error in=w80) -> (error out=w97:errorcluster)  [unwired: 1 out]
              }
              frame True {
              }
            }
            n156 = call-poly <userlib>:"Data Changed__ogtk.vi"("U32"=w62) -> ("Changed"=w61:bool)
            n157 = Not(x=w61) -> (.not. x?=w60:bool)
          }
        }
        n158 = call-dynamic "Delacor_lib_QMH_Error Handler - Helper Loop.vi"("Error Debug"=w49, "error in"=w51, "Message Queue in"=w50) -> ()  [unwired: 7 in, 2 out]
      }
      n159 = Unregister For Events(event registration refnum=w37) -> ()  [unwired: 1 in, 1 out]
      n160 = Unregister For Events(event registration refnum=w33) -> ()  [unwired: 1 in, 1 out]
    }
    frame Error {
      n161 = call "Synchronize Caller Events.vi"("Module Admin"=w336) -> ("Module Admin out"=w335:refnum<class "Delacor_lib_QMH_Cloneable Module Admin.lvclass">)  [unwired: 9 in, 1 out]
      n162 = property on="Property Node" class="Mod Admin"(reference=w335) -> ("Accessors:Module ID"=w334:i32)  [unwired: 1 in, 2 out]
      n163 = call-dynamic "Delacor_lib_QMH_Release Message Queue.vi"("error in"=w342, "Message Queue"=w333) -> ("error out"=w341:errorcluster)  [unwired: 9 in]
      n164 = call "Module Name--constant.vi"("Module ID"=w334) -> ("Module Name"=w339:string)  [unwired: 10 in]
      n165 = Format Into String(format string="An error occurred during initialization. %s is no longer running.", w339) -> (resulting string=w337:string)  [unwired: 2 in, 1 out]
      n166 = call "Error Reported.vi"("Additional Information"=w337, "Error"=w341, "Module ID"=w334) -> ()  [unwired: 8 in, 1 out]
    }
  }
  n167 = Merge Errors(w27, w26) -> (w28:errorcluster)
  n168 = call "Close Module.vi"("error in"=w28, "Wait for stop?"=w14, "Module Admin in"=w16) -> ("error out"=w25:errorcluster, "External Launch"=w13:bool, "Module Admin out"=w15:refnum<class "Delacor_lib_QMH_Cloneable Module Admin.lvclass">)  [unwired: 6 in]
  n169 = Unregister For Events(event registration refnum=w20, error in=w25) -> (error out=w24:errorcluster)
  "error out" <- w24
  n170 = case "External Launch?" shown="True" w13 {
    tunnel: w24 -> [_ w343]
    frame False {
    }
    frame True {
      n171 = case shown="No Error" w343 {
        frame No Error {
          n172 = invoke class="VI" method="FP.Close"() -> ()  [unwired: 3 in, 3 out]
        }
        frame Error {
          n173 = disable-structure shown="Default" {
            frame condition #0 (active) {
              n174 = invoke class="VI" method="FP.Open"("Activate"=TRUE ("Activate?")) -> ()  [unwired: 4 in, 5 out]
            }
            frame condition #1 {
              # "Don't show panel on error if running inside a built EXE."
            }
          }
        }
      }
    }
  }
  n175 = local write "Module Admin"(w15) -> ()
